vi "例7.8强度图.vi"() -> ()   [LabVIEW 2017]
panel:
  out "二维数组":i32[][](array[numeric])
  out "强度图":i32[][](graph)
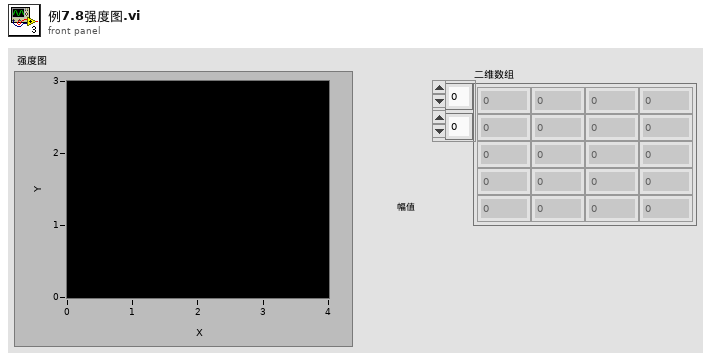
[diagram p1: front panel]
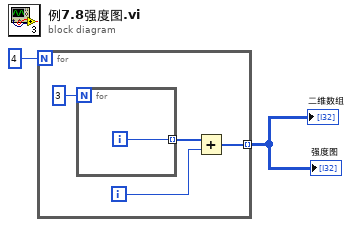
[diagram p0: block diagram]
diagram:
  n1 = for {
    N: 4 -> [_]
    tunnel: [w4] -> w2 mode=indexing
    i -> [w3]
    n2 = for {
      N: 3 -> [_]
      tunnel: [w7] -> w5 mode=indexing
      i -> [w7]
    }
    n3 = Add(x=w5, y=w3) -> (x+y=w4:i32[])
  }
  "强度图" <- w2
  "二维数组" <- w2
